vi "Get Operator and Location.vi"() -> (3 "Meta Data":T1)   [LabVIEW 2019]
doc: "Simple Dialog Box that returns the operator name and calibration location as two strings."
panel:
  in  "Comments":string
  in  "Cal Tube SN":string
  in  "Sensor SN":string
  out "error out":errorcluster
  in  "OK Button":bool
  in  "Calibration Location":string
  in  "Operator Name":string
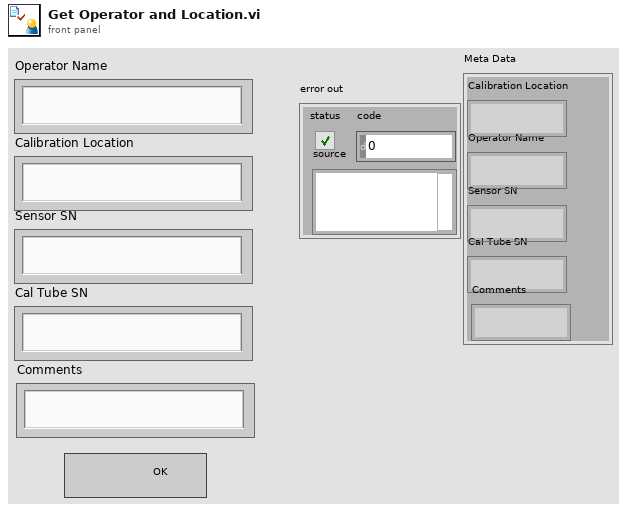
[diagram p1: front panel]
types:
  T1 = cluster{"Calibration Location":string, "Operator Name":string, "Sensor SN":string, "Cal Tube SN":string, "Comments":string}
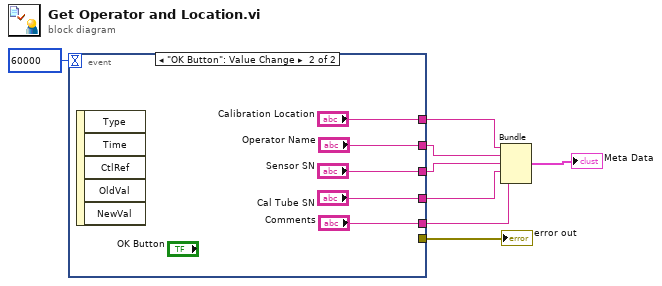
[diagram p0: block diagram]
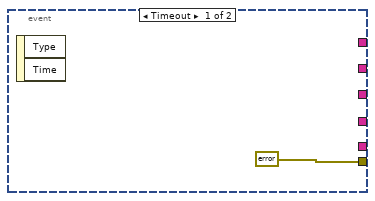
[diagram p2: hidden frame]
diagram:
  n1 = event shown="[1] \"OK Button\": Value Change" {
    selector: _ -> [_ _]
    dyn-events: _ -> [_ _]
    timeout: 60000 -> [_ _]
    tunnel: [errorcluster {"status"=TRUE, "code"=0, "source"="Needed to Enter Operator/Location"} ("error constant") _] -> w7
    tunnel: [_ "Calibration Location"] -> w6
    tunnel: [_ "Operator Name"] -> w5
    tunnel: [_ "Sensor SN"] -> w4
    tunnel: [_ "Cal Tube SN"] -> w3
    tunnel: [_ "Comments"] -> w1
    event Timeout {
      n2 = event-data() -> ()  [unwired: 1 in, 2 out]
    }
    event "OK Button": Value Change {
      n3 = event-data() -> ()  [unwired: 1 in, 5 out]
    }
  }
  "error out" <- w7
  n4 = Bundle("Calibration Location"=w6, "Operator Name"=w5, "Sensor SN"=w4, "Cal Tube SN"=w3, "Comments"=w1) -> (→"Meta Data":T1)  [unwired: 1 in]
